vi "backup current calibration data.vi"(8 "error in (no error)":errorcluster) -> (0 "error out":errorcluster, 3 "backup file path":path)   [LabVIEW 2020]
panel:
  out "Application Directory":path
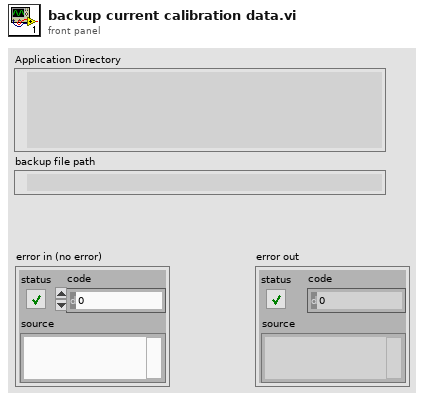
[diagram p1: front panel]
types:
  T1 = enum16{"Initialise", "Load from file", "Save to file", "Read", "Write"}
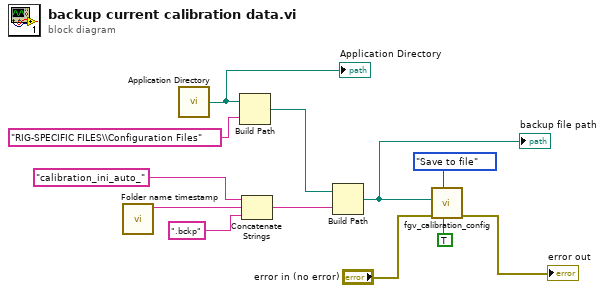
[diagram p0: block diagram]
diagram:
  n1 = call "Folder name timestamp.vi"() -> ("date/time string"=w8:string)  [unwired: 11 in]
  n2 = call <vilib>:"Application Directory.vi"() -> ("Application Directory"=w12:path)
  "Application Directory" <- w12
  n3 = Build Path(base path=w12, name or relative path="RIG-SPECIFIC FILES\\Configuration Files") -> (appended path=w6:path)
  n4 = Concatenate Strings("calibration_ini_auto_" ("string"), w8, ".bckp" ("string")) -> (w9:string)
  n5 = Build Path(base path=w6, name or relative path=w9) -> (appended path=w3:path)
  "backup file path" <- w3
  n6 = call "fgv_calibration_config.vi"("Non default file path?"=TRUE, "Cal config ops"=T1."Save to file", "error in (no error)"="error in (no error)", "config file path"=w3) -> ("error out"=→"error out":errorcluster)  [unwired: 5 in, 2 out]
